vi "Read TX.Data.vi"(8 "error in (no error)":errorcluster, 11 "Devices in":refnum<class "Devices.lvclass">) -> (0 "error out":errorcluster, 2 "TX.Data":T1 caption="Transmission Data" format="%.0x", 3 "Devices out":refnum<class "Devices.lvclass">)   [LabVIEW 2020, in "Devices.lvclass"]
uses:
  Devices.lvclass
  TypeDef/Transmission Data.ctl
  Devices.lvclass/Devices.ctl
  I2C Controller Lib.lvlib
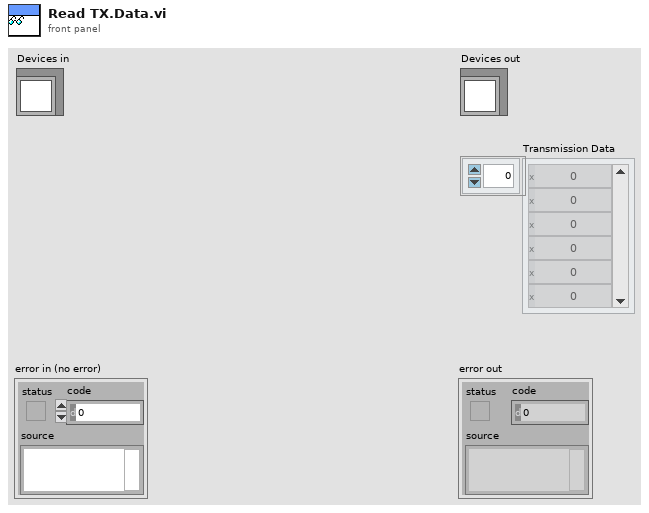
[diagram p1: front panel]
types:
  T1 = typedef "I2C Controller Lib.lvlib/Transmission Data.ctl" = u8[]
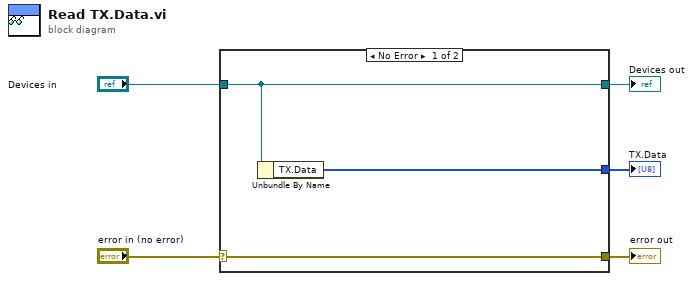
[diagram p0: block diagram]
diagram:
  n1 = case shown="No Error" "error in (no error)" {
    selector: "error in (no error)" -> [w8 w9]
    tunnel: [w8 w9] -> w4
    tunnel: [w7 w10] -> w2
    tunnel: "Devices in" -> [w7 w10]
    tunnel: [w6 _] -> w1
    frame No Error {
      n2 = Unbundle By Name(w7) -> ("TX.Data"=w6:T1)
    }
    frame Error {
    }
  }
  "error out" <- w4
  "Devices out" <- w2
  "TX.Data" <- w1
